vi "sinanju_getPos.vi"(0 "连接ID":refnum<k5>, 1 "错误输入（无错误）":errorcluster) -> (2 "连接ID输出":refnum<k5>, 3 "错误输出":errorcluster, 4 "值":sgl, 5 "值 2":sgl, 6 "值 3":sgl, 7 "值 4":sgl)   [LabVIEW 2017]
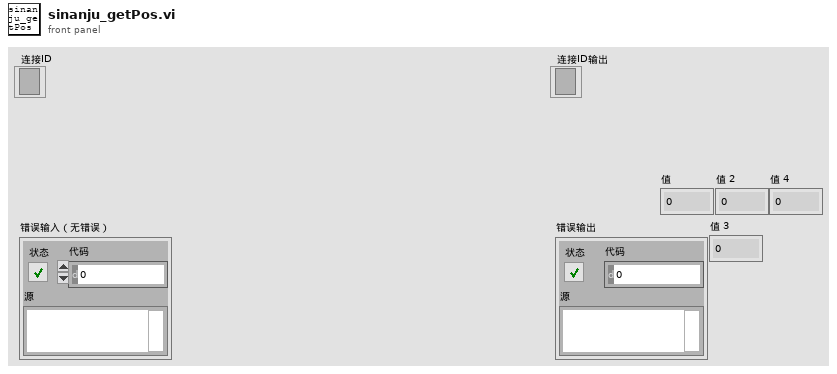
[diagram p1: front panel]
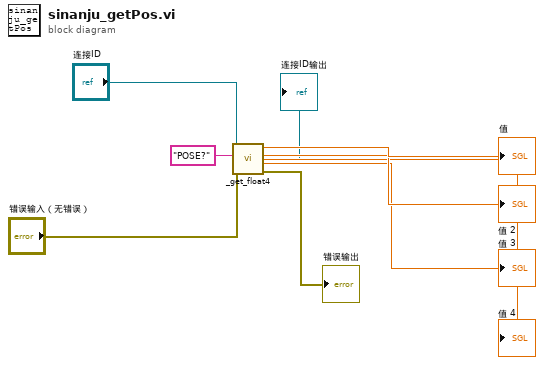
[diagram p0: block diagram]
diagram:
  n1 = call "_get_float4.vi"("错误输入（无错误）"="错误输入（无错误）", "写入缓冲区"="POSE?", "连接ID"="连接ID") -> ("错误输出"=→"错误输出":errorcluster, "值 3"=→"值 3":sgl, "值 2"=→"值 2":sgl, "值"=→"值":sgl, "值 4"=→"值 4":sgl, "连接ID输出"=→"连接ID输出":refnum<k5>)  [unwired: 1 in]
